vi "Test Subvi.vi"(10 "Slide":dbl(slide) scale=0.0..10.0) -> (2 "Numeric 2":dbl)   [LabVIEW 2012]
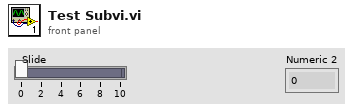
[diagram p1: front panel]
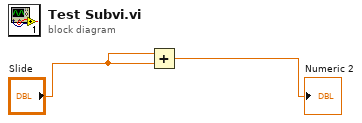
[diagram p0: block diagram]
diagram:
  n1 = Add(x="Slide", y="Slide") -> (x+y=→"Numeric 2":dbl)
